vi "SolveIKPosition.vi"(4 "error in":errorcluster, 5 "Pose":T2={"Position"={"x"=0.457, "y"=-0.385, "z"=-0.261}, "Orientation"={"Roll (y)"=3.13, "Pitch (x)"=-0.1, "Yaw (z)"=-1.85}}, 6 "Side":T3, 7 "node":string) -> (0 "error out":errorcluster)   [LabVIEW 2012]
doc: "Solve inverse kinematics problem based on a given pose"
uses:
  <userlib>/ROSforLV/ROS/Code/SubVIs/BaxterSide.ctl
  <userlib>/ROSforLV/ROS/Code/Console/Servers/ServerSubs/TopicDef.ctl
  <userlib>/ROSforLV/ROS/Code/SubVIs/_ROSDirection.ctl
  <userlib>/ROSforLV/ROS/MessageBuilding/std_msgs/subs/u32Scalar.vi
panel:
  out "IK Reply":T1
  out "Reply":string
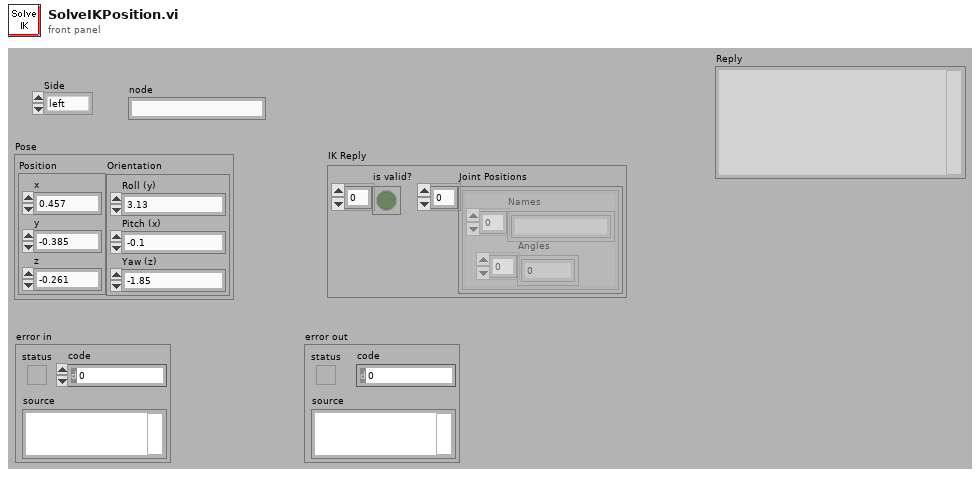
[diagram p1: front panel]
types:
  T1 = cluster{"is valid?":bool[], "Joint Positions":cluster{"Angles":dbl[], "Names":string[]}[]}
  T2 = cluster{"Position":cluster{"x":dbl, "y":dbl, "z":dbl}, "Orientation":cluster{"Roll (y)":dbl, "Pitch (x)":dbl, "Yaw (z)":dbl}}
  T3 = typedef "BaxterSide.ctl" = enum16{"left", "right"}
  T4 = typedef "TopicDef.ctl" = cluster{"Topic":string, "Type":string, "Action":T5, "Update (ms)":u16, "queue size":u16}
  T5 = typedef "_ROSDirection.ctl" = enum16{"Node", "Publisher", "Subscriber", "ServiceClient", "ServiceProvider"}
  T6 = cluster{"Roll (y)":dbl, "Pitch (x)":dbl, "Yaw (z)":dbl}
  T7 = typedef "_ROSControl.ctl" = cluster{"topic port":u16, "Node":string, "topic":string, "type":string, "node port":u16, "error ":errorcluster, "Direction":T5, "Update (ms)":u16, "FIFO size":u16}
  T8 = cluster{"Position":cluster{"x":dbl, "y":dbl, "z":dbl}, "Quaternion":cluster{"x":dbl, "y":dbl, "z":dbl, "w":dbl}}
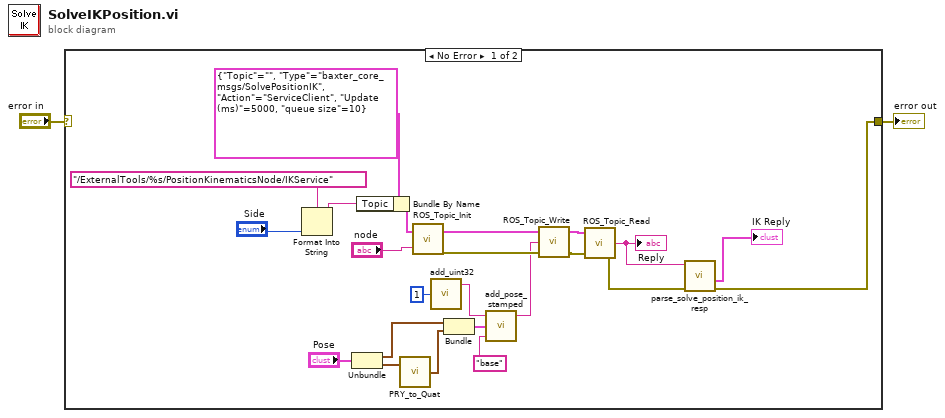
[diagram p0: block diagram]
diagram:
  n1 = case shown="No Error" "error in" {
    selector: "error in" -> [_ w26]
    tunnel: [w3 w26] -> w2
    frame No Error {
      n2 = Format Into String(format string="/ExternalTools/%s/PositionKinematicsNode/IKService" ("topic"), "Side") -> (resulting string=w12:string)  [unwired: 2 in, 1 out]
      n3 = Unbundle("Pose") -> ("Position"=w21:cluster{"x":dbl, "y":dbl, "z":dbl}, "Orientation"=w23:T6)
      n4 = Bundle By Name(cluster=T4 {"Topic"="", "Type"="baxter_core_msgs/SolvePositionIK", "Action"=enum."ServiceClient", "Update (ms)"=5000, "queue size"=10} ("Definitions"), "Topic"=w12) -> (w8:T4)
      n5 = call <userlib>:"PRY_to_Quat.vi"("Orientation"=w23) -> ("Quaternion"=w22:cluster{"x":dbl, "y":dbl, "z":dbl, "w":dbl})  [unwired: 1 in]
      n6 = call <userlib>:"ROS_Topic_Init.vi"("node"="node", "Definitions"=w8) -> ("error out"=w6:errorcluster, "ROS out"=w16:T7)
      n7 = call-poly <userlib>:"add_uint32.vi"("Numeric"=u32 1) -> ("msg out"=w17:string)  [unwired: 4 in]
      n8 = Bundle("Position"=w21, "Quaternion"=w22) -> (w20:T8)  [unwired: 1 in]
      n9 = call <userlib>:"add_pose_stamped.vi"("frame_id"="base", "Pose"=w20, "msg in"=w17) -> ("msg out"=w5:string)  [unwired: 2 in]
      n10 = call <userlib>:"ROS_Topic_Write.vi"("error in (no error)"=w6, "Msg in"=w5, "ROS in"=w16) -> ("error out"=w7:errorcluster, "ROS out"=w13:T7)  [unwired: 1 in]
      n11 = call <userlib>:"ROS_Topic_Read.vi"("error in (no error)"=w7, "ROS in"=w13) -> ("error out"=w4:errorcluster, "Reply"=w15:string)  [unwired: 1 in, 1 out]
      "Reply" <- w15
      n12 = call <userlib>:"parse_solve_position_ik_resp.vi"("error in"=w4, "msg in"=w15) -> ("error out"=w3:errorcluster, "IK Reply"=→"IK Reply":T1)  [unwired: 2 in, 2 out]
    }
    frame Error {
    }
  }
  "error out" <- w2
